vi "class_data.vi"() -> ()   [LabVIEW 2010, in "FPGAWrapperDL090211Galvo.lvclass"]
uses:
  FPGAWrapperDL090211Galvo.lvclass
  type definitions/settings_cluster.ctl
  common_typedefs/channels_cluster.ctl
  type definitions/gate_cluster.ctl
  common_typedefs/gate_parameters_cluster.ctl
panel:
  in  "settings writer endpoint":refnum<k21>
  in  "data reader endpoint":refnum<k21>
  in  "command writer endpoint":refnum<k21>
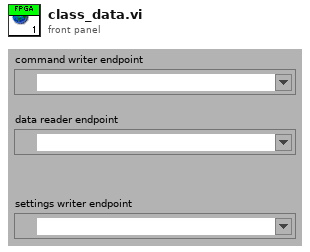
[diagram p1: front panel]
diagram:
